vi "Create Controller.vi"(8 "error in (no error)":errorcluster, 11 "AI Driver":refnum<class "AI Driver.lvclass">[](array[class])) -> (0 "error out":errorcluster, 3 "DAQ Controller out":refnum<class "DAQ Controller.lvclass">)   [LabVIEW 2022 SP3, in "DAQ Controller.lvclass"]
uses:
  DAQ Controller.lvclass
  AI Driver/AI Driver.lvclass
  DAQ Actor/DAQ Actor/DAQ Process.lvclass
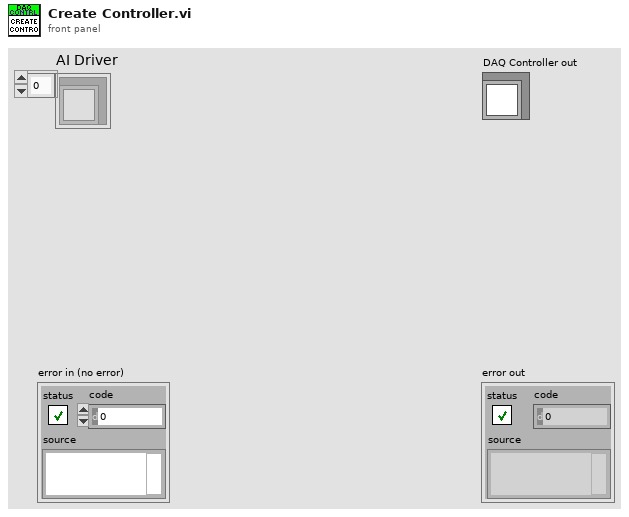
[diagram p1: front panel]
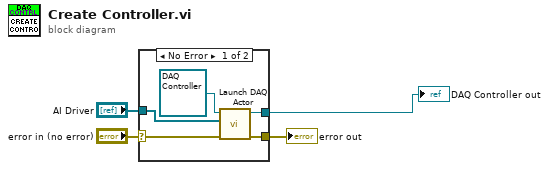
[diagram p0: block diagram]
diagram:
  n1 = case shown="No Error" "error in (no error)" {
    selector: "error in (no error)" -> [w7 w10]
    tunnel: [w6 w10] -> w3
    tunnel: "AI Driver" -> [w9 _]
    tunnel: [w5 _] -> w1
    frame No Error {
      n2 = call "Launch DAQ Actor.vi"("error in (no error)"=w7, "AI Driver"=w9, "DAQ Controller"=refnum<class "DAQ Controller.lvclass"> refnum ("DAQ Controller in")) -> ("error out"=w6:errorcluster, "DAQ Controller"=w5:refnum<class "DAQ Controller.lvclass">)  [unwired: 7 in]
    }
    frame Error {
    }
  }
  "error out" <- w3
  "DAQ Controller out" <- w1
